vi "Variant Loader.vi"(6 "error in (no error)":errorcluster, 9 "TS UI Data out":T1) -> (0 "error out":errorcluster, 3 "TS UI Data out":T1)   [LabVIEW 2015]
uses:
  <vilib>/Utility/config.llb/NI_LVConfig.lvlib
  Type defs/Variant Loader States.ctl
  Type defs/TS UI Data.ctl
  Type defs/Nest cluster.ctl
panel:
  in  "Load Button":bool
  in  "Part Number":string
  in  "Description":string
  in  "Variant":string(combo)
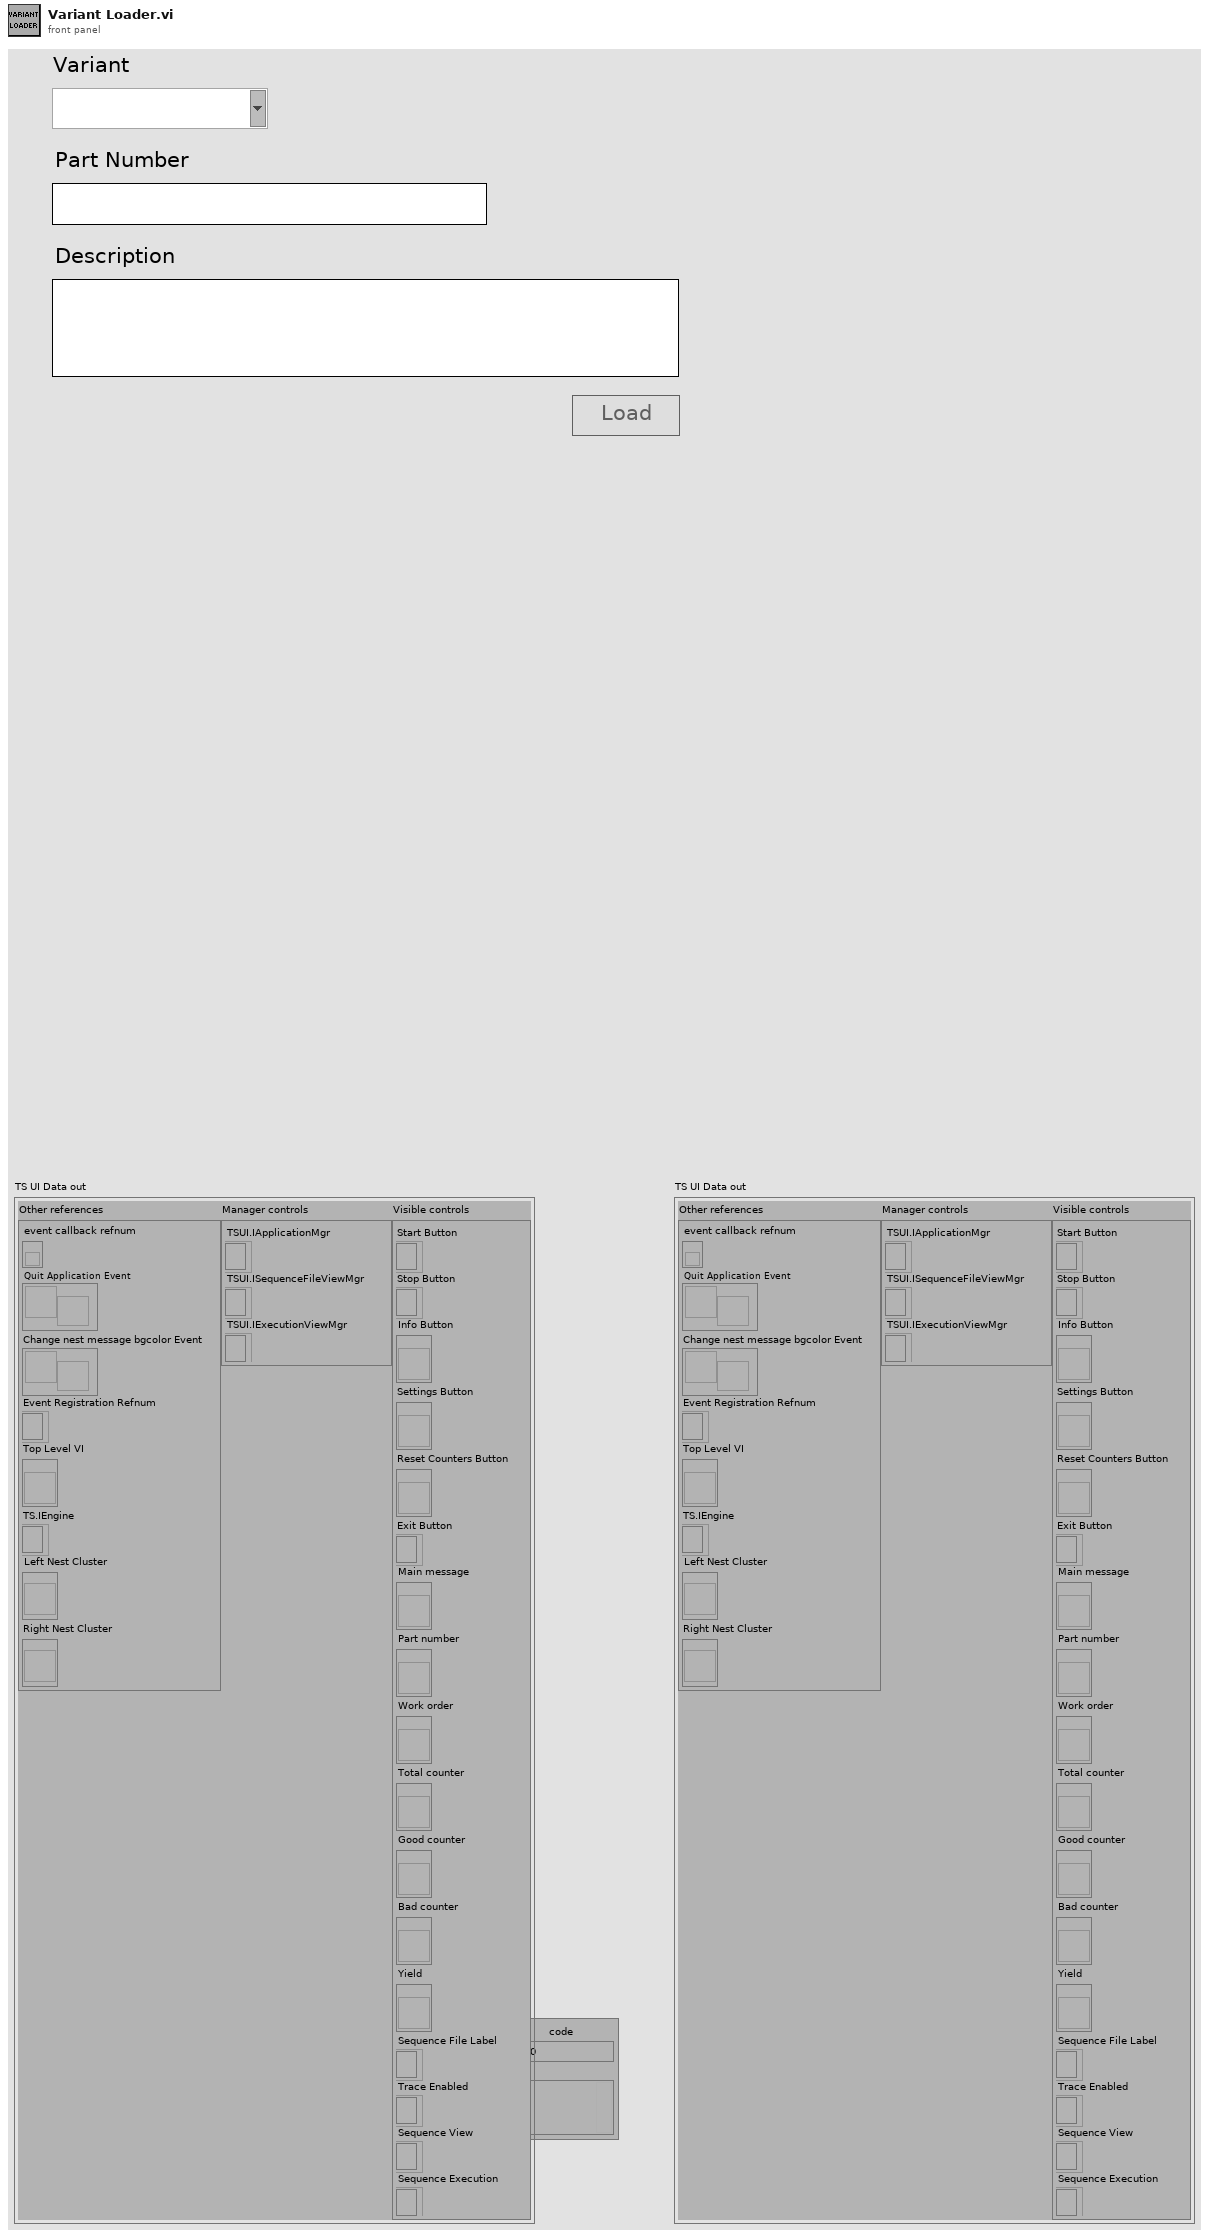
[diagram p1: front panel]
types:
  T1 = typedef "TS UI Data.ctl" = cluster{"Other references":cluster{"event callback refnum":refnum<k27>, "Quit Application Event":refnum<user-event>, "Change nest message bgcolor Event":refnum<user-event>, "event registration refnum":refnum<event-registration>, "Top Level VI":refnum<vi>, "TS.IEngine":refnum<k7>, "Left Nest Cluster":refnum<vi>, "Right Nest Cluster":refnum<vi>}, "Manager controls":cluster{"TSUI.IApplicationMgr":refnum<k7>, "TSUI.ISequenceFileViewMgr":refnum<k7>, "TSUI.IExecutionViewMgr":refnum<k7>}, "Visible controls":cluster{"Start Button":refnum<k7>, "Stop Button":refnum<k7>, "Info Button":refnum<vi>, "Settings Button":refnum<vi>, "Reset Counters Button":refnum<vi>, "Exit Button":refnum<k7>, "Main message":refnum<vi>, "Part number":refnum<vi>, "Work order":refnum<vi>, "Total counter":refnum<vi>, "Good counter":refnum<vi>, "Bad counter":refnum<vi>, "Yield":refnum<vi>, "Sequence File Label":refnum<k7>, "Trace Enabled":refnum<k7>, "Sequence View":refnum<k7>, "Sequence Execution":refnum<k7>}}
  T2 = typedef "Variant Loader States.ctl" = enum16{"Init", "Get Variants", "Load Variant Data", "Event Handler", "Exit"}
  T3 = enum8{"Enabled", "Disabled", "Disabled and Grayed Out"}
  T4 = typedef "NI_LVConfig.lvlib/Config Data RefNum.ctl" = refnum<k1>
  T5 = typedef "Variant Data Cluster.ctl" = cluster{"Program":string, "Description":string, "PN Customer":string, "Variant":string, "Customer FW Folder":string, "File":string, "Total Units":string, "Good Units":string, "Bad Units":string, "Yield":string}
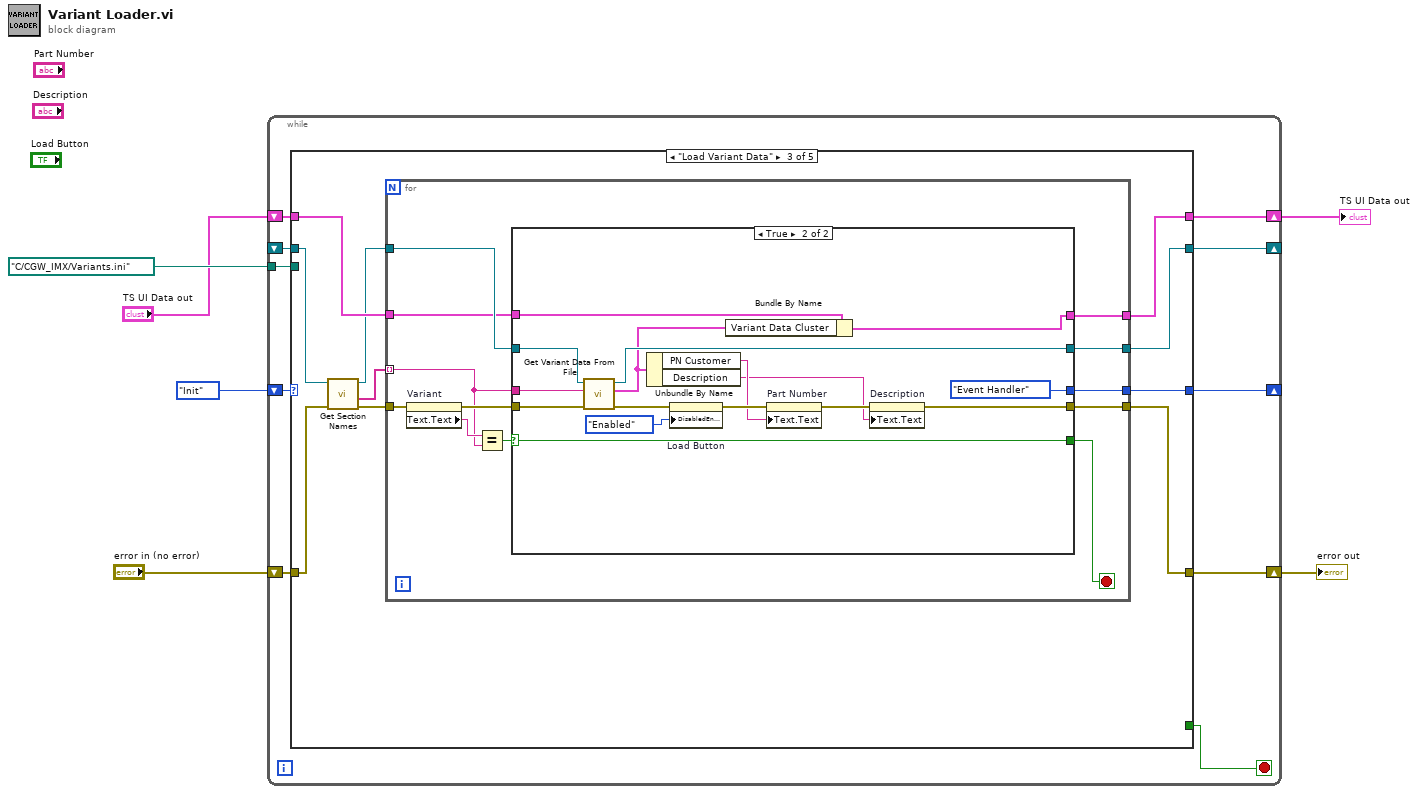
[diagram p0: block diagram]
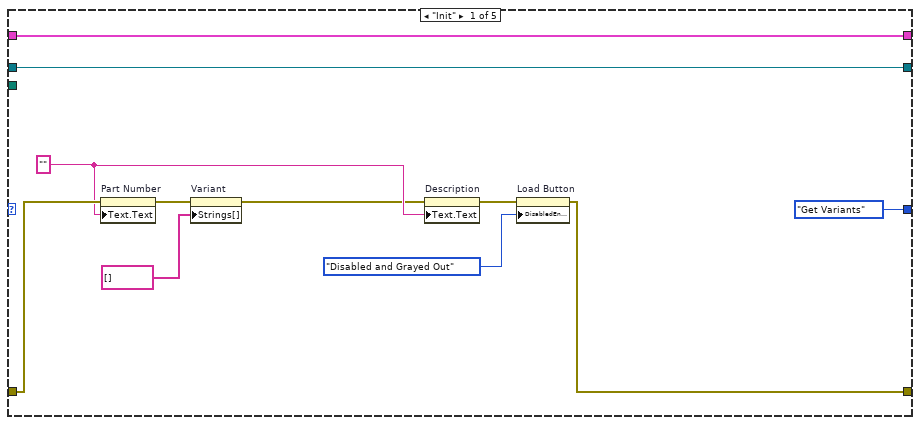
[diagram p2: hidden frame]
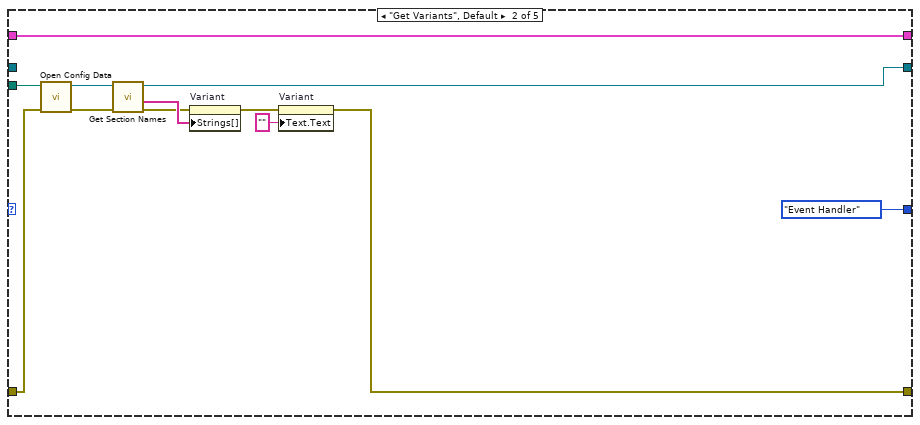
[diagram p3: hidden frame]
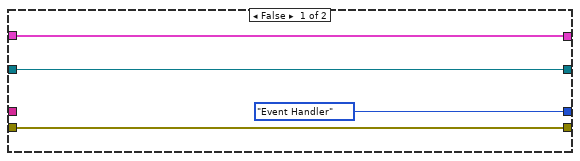
[diagram p4: hidden frame]
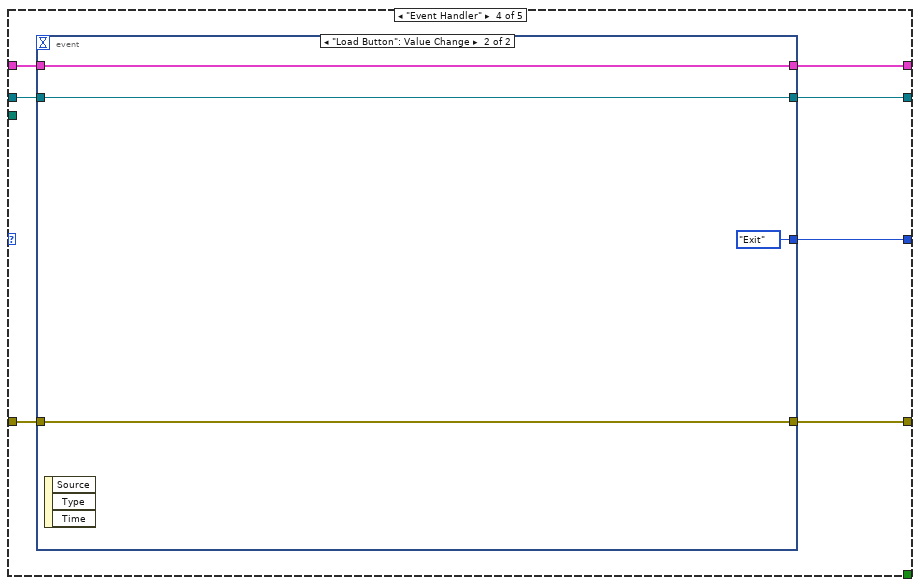
[diagram p5: hidden frame]
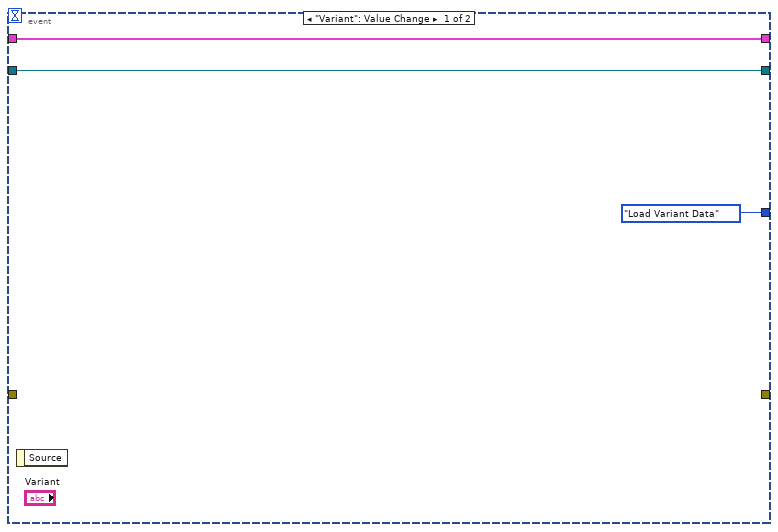
[diagram p6: hidden frame]
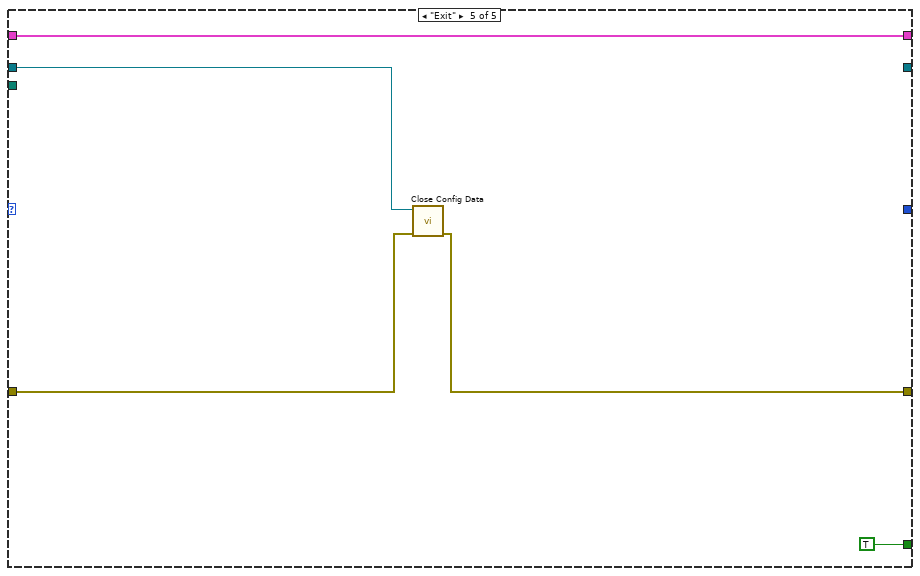
[diagram p7: hidden frame]
diagram:
  n1 = while {
    tunnel: path "C:/CGW_IMX/Variants.ini" ("configuration file path") -> [w16]
    shift-right: [w13] -> _
    shift-left: Variant_Loader_States."Init" -> [w14]
    shift-right: [w11] -> _
    shift-left: _ -> [w12]
    shift-right: [w7] -> w1
    shift-left: "TS UI Data out" -> [w10]
    shift-right: [w9] -> w2
    shift-left: "error in (no error)" -> [w15]
    stop <- w8 stop-if-true
    n2 = case shown="\"Load Variant Data\"" w14 {
      tunnel: w16 -> [_ w39 _ _ _]
      tunnel: w15 -> [w27 w34 w49 w88 w99]
      tunnel: [w21 w28 w45 w82 w98] -> w9
      tunnel: [Variant_Loader_States."Get Variants" Variant_Loader_States."Event Handler" w43 w87 _] -> w13
      tunnel: [w20 w32 w44 w85 _] -> w11
      tunnel: w12 -> [w20 _ w42 w86 w97]
      tunnel: w10 -> [w19 w31 w46 w84 w96]
      tunnel: [_ _ _ _ TRUE] -> w8
      tunnel: [w19 w31 w40 w83 w96] -> w7
      frame "Init" {
        w18 = ""
        n3 = property on="Part Number" class="Str"(error in=w27, "Text.Text"=w18) -> (error out=w26:errorcluster)  [unwired: 1 in, 1 out]
        n4 = property on="Variant" class="CmbBox"(error in=w26, "Strings[]"=string[] [] ("Strings []")) -> (error out=w17:errorcluster)  [unwired: 1 in, 1 out]
        n5 = property on="Description" class="Str"(error in=w17, "Text.Text"=w18) -> (error out=w23:errorcluster)  [unwired: 1 in, 1 out]
        n6 = property on="Load Button" class="Bool"(error in=w23, "DisabledEnum"=T3."Disabled and Grayed Out" ("Disabled")) -> (error out=w21:errorcluster)  [unwired: 1 in, 1 out]
      }
      frame "Get Variants", Default {
        n7 = call <vilib>:"Open Config Data.vi"("error in (no error)"=w34, "configuration file path"=w39) -> ("error out"=w37:errorcluster, "refnum"=w38:T4)  [unwired: 7 in, 1 out]
        n8 = call <vilib>:"Get Section Names.vi"("error in (no error)"=w37, "refnum"=w38) -> ("error out"=w35:errorcluster, "section names"=w36:string[], "refnum out"=w32:T4)  [unwired: 7 in]
        n9 = property on="Variant" class="CmbBox"(error in=w35, "Strings[]"=w36) -> (error out=w30:errorcluster)  [unwired: 1 in, 1 out]
        n10 = property on="Variant" class="CmbBox"(error in=w30, "Text.Text"="") -> (error out=w28:errorcluster)  [unwired: 1 in, 1 out]
      }
      frame "Load Variant Data" {
        n11 = call <vilib>:"Get Section Names.vi"("error in (no error)"=w49, "refnum"=w42) -> ("error out"=w47:errorcluster, "section names"=w48:string[], "refnum out"=w41:T4)  [unwired: 7 in]
        n12 = for {
          tunnel: w48 -> [w56] mode=indexing
          tunnel: w47 -> [w60]
          tunnel: w46 -> [w52]
          tunnel: w41 -> [w55]
          tunnel: [w57] -> w45
          tunnel: [w54] -> w44
          tunnel: [w53] -> w43
          tunnel: [w51] -> w40
          stop <- w50 stop-if-true
          n13 = property on="Variant" class="CmbBox"(error in=w60) -> (error out=w58:errorcluster, "Text.Text"=w61:string)  [unwired: 1 in, 1 out]
          n14 = Equal?(x=w61, y=w56) -> (x = y?=w59:bool)
          n15 = case shown="True" w59 {
            selector: w59 -> [_ w74]
            tunnel: w58 -> [w65 w81]
            tunnel: [w65 w71] -> w57
            tunnel: w56 -> [_ w80]
            tunnel: w55 -> [w64 w79]
            tunnel: [w64 w78] -> w54
            tunnel: [Variant_Loader_States."Event Handler" Variant_Loader_States."Event Handler"] -> w53
            tunnel: w52 -> [w62 w68]
            tunnel: [w62 w67] -> w51
            tunnel: [_ w74] -> w50
            frame False {
            }
            frame True {
              n16 = call "Get Variant Data From File.vi"("error in (no error)"=w81, "Variant Name"=w80, "File refnum in"=w79) -> ("error out"=w76:errorcluster, "Variant Data Cluster"=w66:T5, "File refnum out"=w78:T4)  [unwired: 6 in]
              n17 = Unbundle By Name(w66) -> ("PN Customer"=w70:string, "Description"=w69:string)
              n18 = property on="Load Button" class="Bool"(error in=w76, "DisabledEnum"=T3."Enabled" ("Disabled")) -> (error out=w73:errorcluster)  [unwired: 1 in, 1 out]
              n19 = Bundle By Name(cluster=w68, "Variant Data Cluster"=w66) -> (w67:T1)
              n20 = property on="Part Number" class="Str"(error in=w73, "Text.Text"=w70) -> (error out=w72:errorcluster)  [unwired: 1 in, 1 out]
              n21 = property on="Description" class="Str"(error in=w72, "Text.Text"=w69) -> (error out=w71:errorcluster)  [unwired: 1 in, 1 out]
            }
          }
        }
      }
      frame "Event Handler" {
        n22 = event shown="[1] \"Load Button\": Value Change" {
          selector: _ -> [_ _]
          dyn-events: _ -> [_ _]
          timeout: _ -> [_ _]
          tunnel: w88 -> [_ w93]
          tunnel: [Variant_Loader_States."Load Variant Data" Variant_Loader_States."Exit"] -> w87
          tunnel: w86 -> [w90 w92]
          tunnel: [w90 w92] -> w85
          tunnel: w84 -> [w89 w94]
          tunnel: [w89 w94] -> w83
          tunnel: [_ w93] -> w82
          event "Variant": Value Change {
            n23 = event-data() -> ()  [unwired: 1 in, 1 out]
          }
          event "Load Button": Value Change {
            n24 = event-data() -> ()  [unwired: 1 in, 3 out]
          }
        }
      }
      frame "Exit" {
        n25 = call <vilib>:"Close Config Data.vi"("error in (no error)"=w99, "refnum"=w97) -> ("error out"=w98:errorcluster)  [unwired: 8 in, 1 out]
      }
    }
  }
  "error out" <- w2
  "TS UI Data out" <- w1
